vi "Calculate_Trace_Variables.vi"(8 "Baseline":i16, 9 "Threshold":u16, 10 "Peak threshold":i16, 11 "Data in":u16[](array[numeric])) -> (0 "Offset":i16, 1 "Pulse height":i16, 2 "Cut off":i16, 3 "Number of peaks":i16, 4 "Integral":i32, 5 "Data out":u16[](array[numeric]))   [LabVIEW 2013]
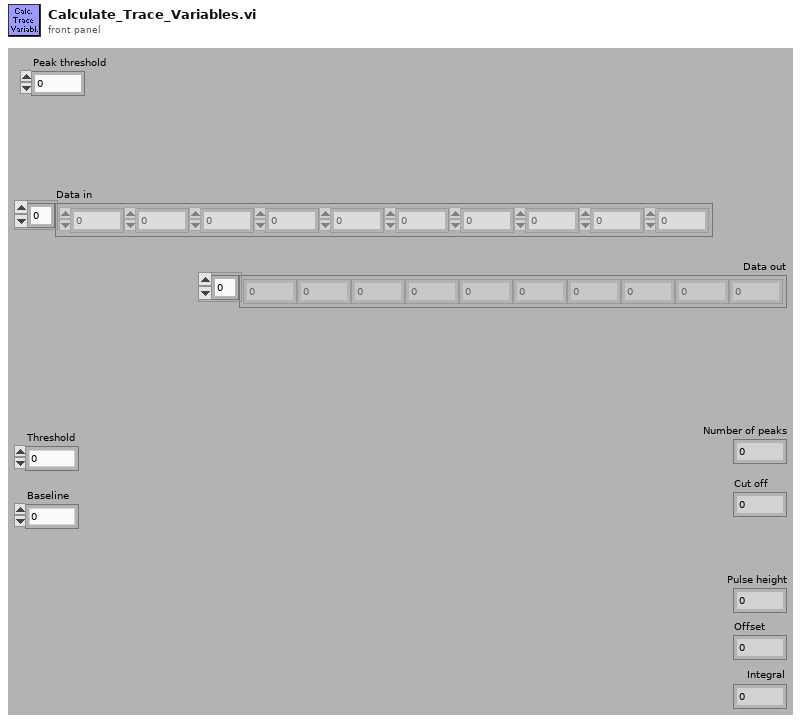
[diagram p1: front panel]
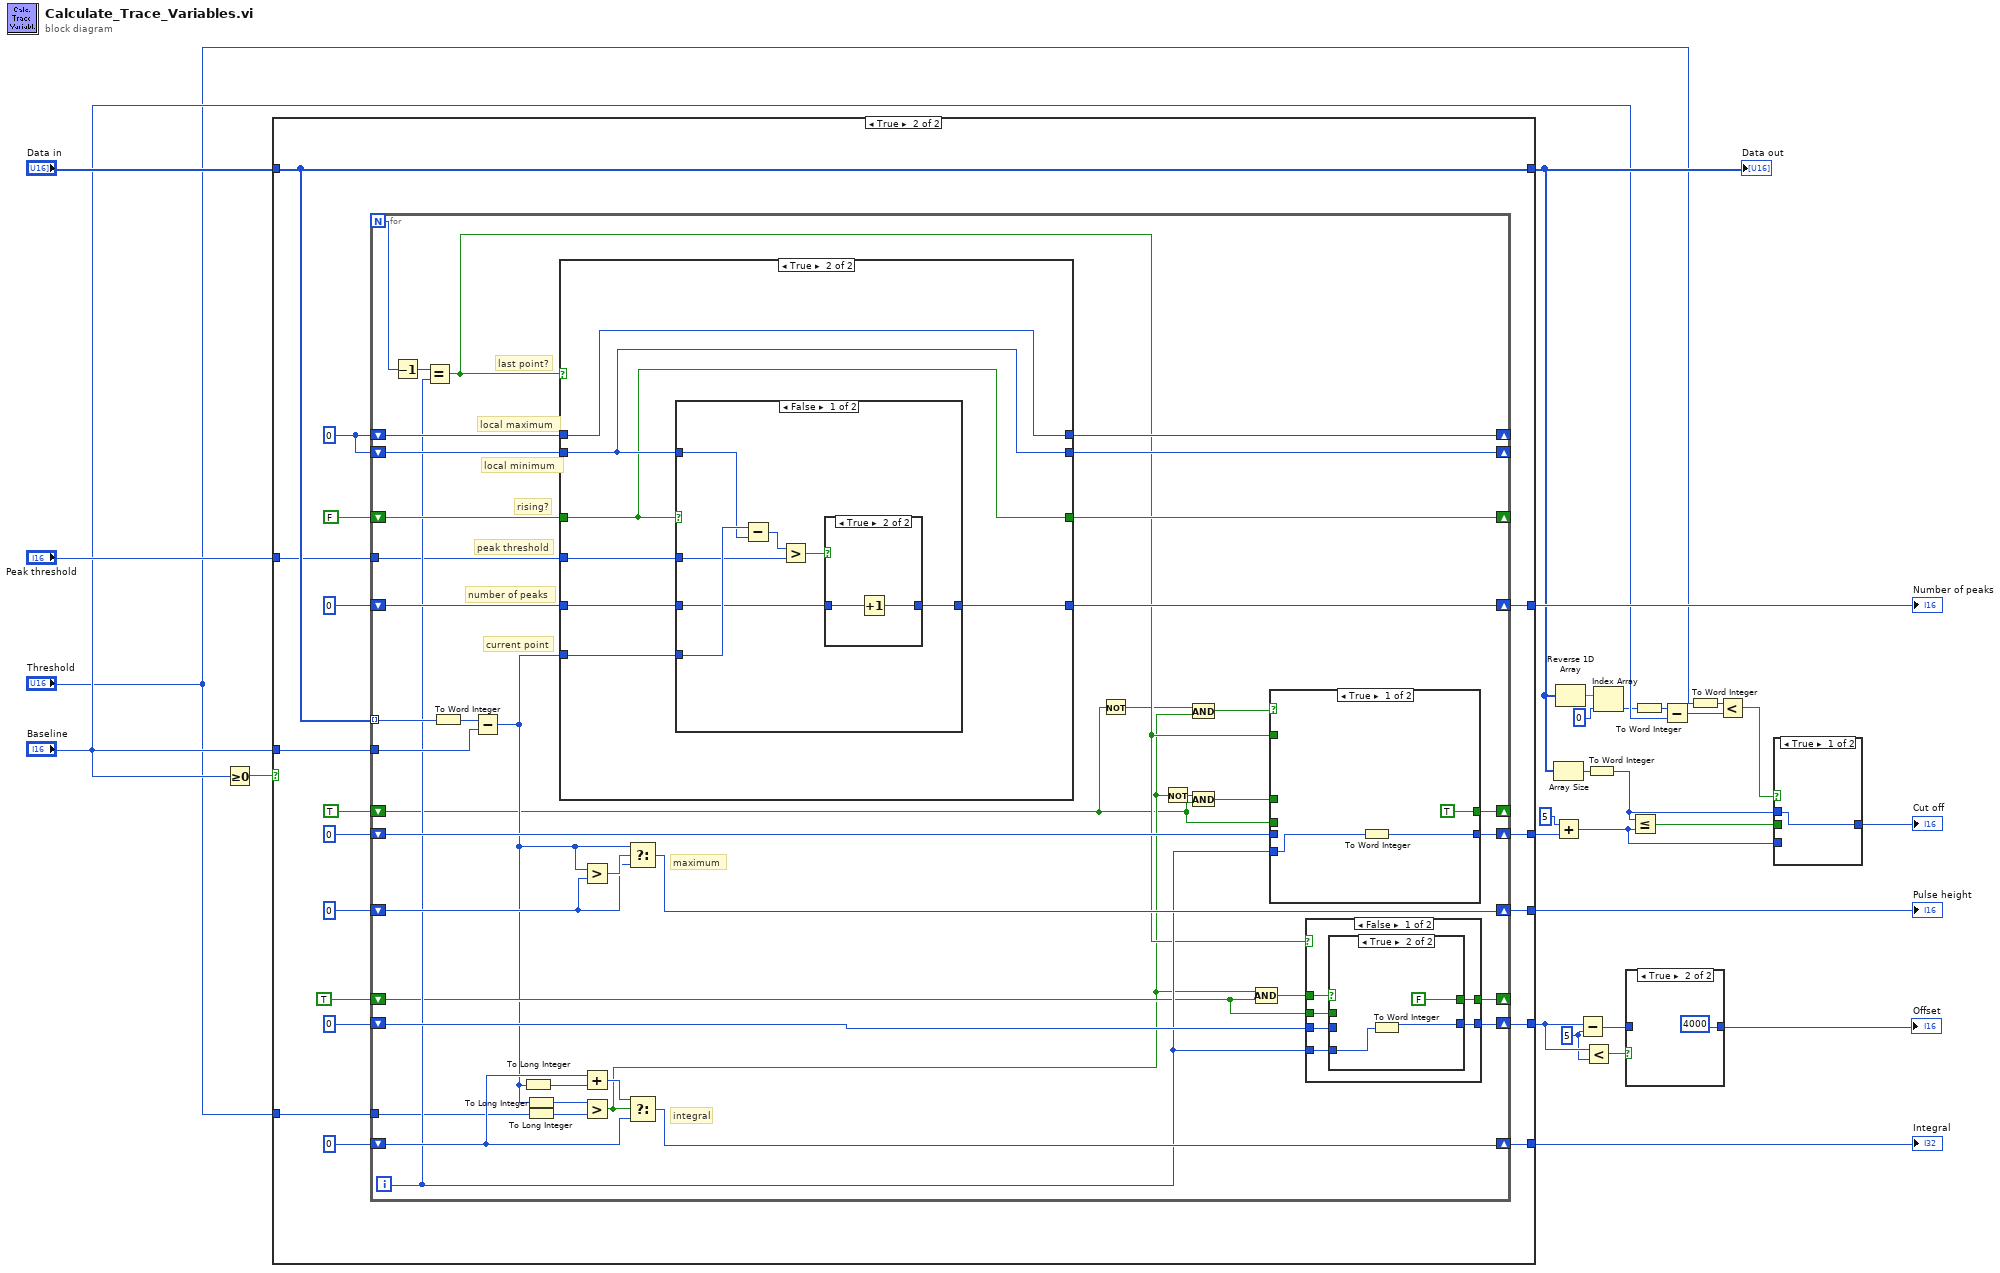
[diagram p0: block diagram]
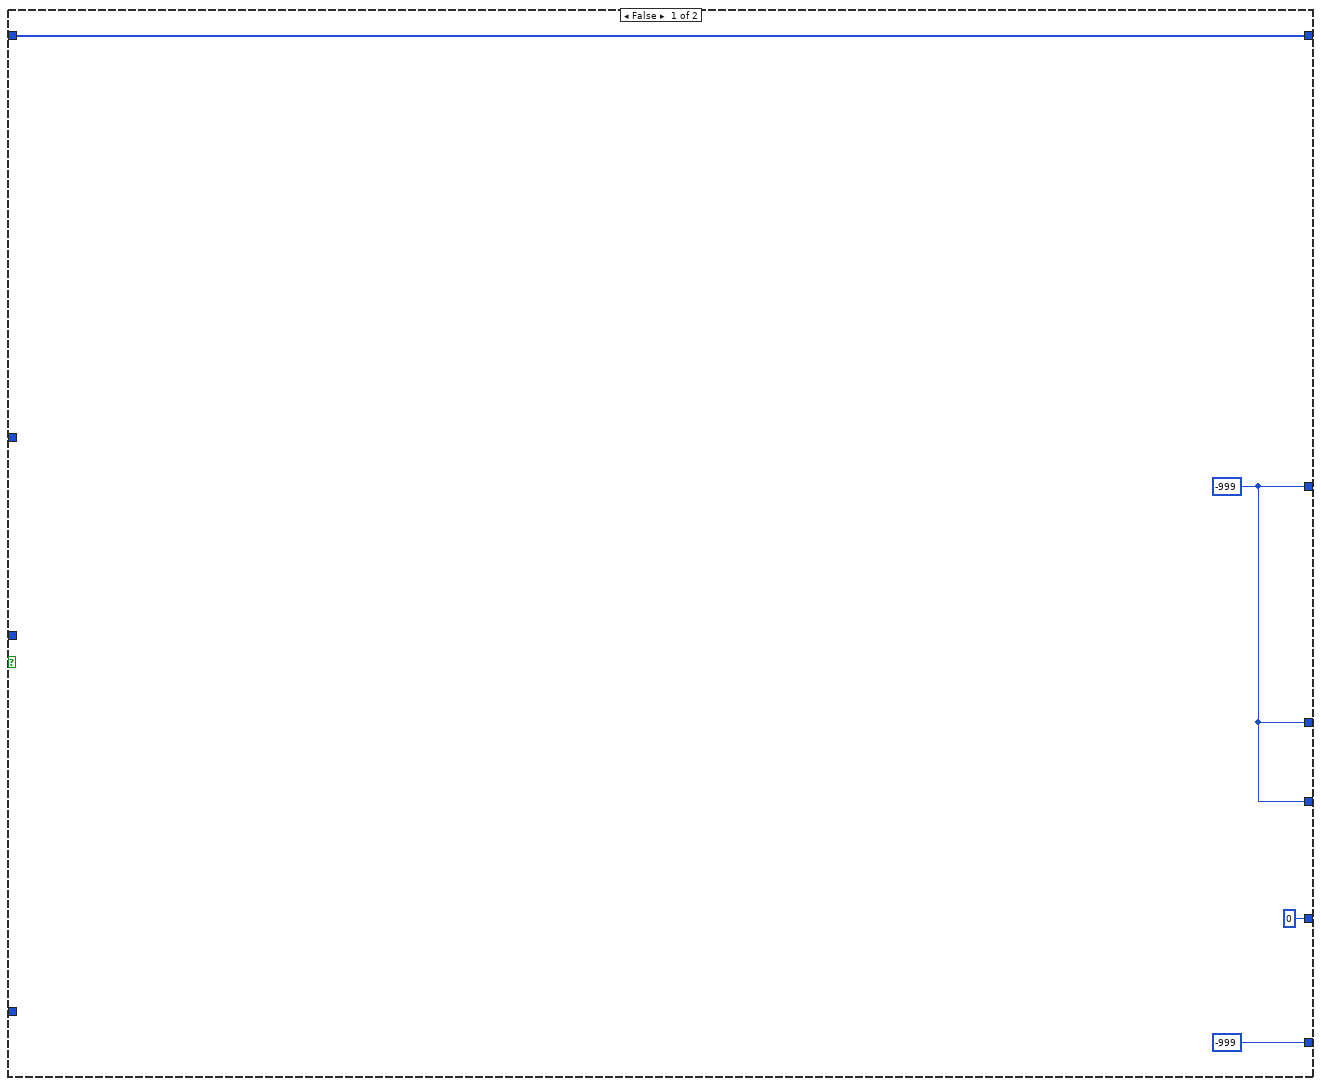
[diagram p5: hidden frame]
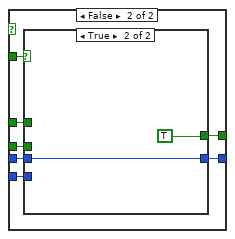
[diagram p6: hidden frame]
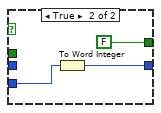
[diagram p8: hidden frame]
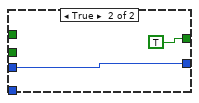
[diagram p10: hidden frame]
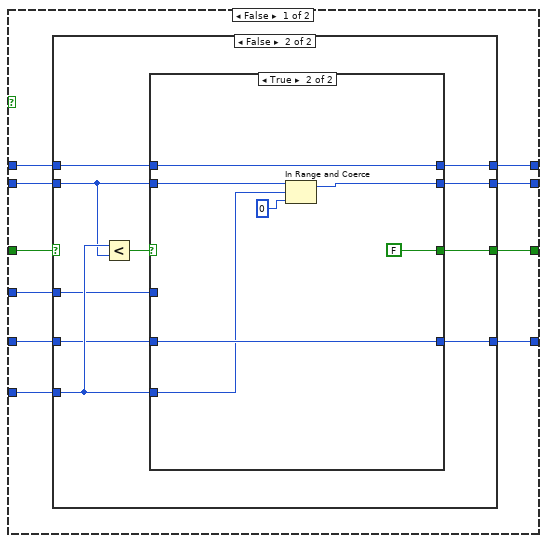
[diagram p11: hidden frame]
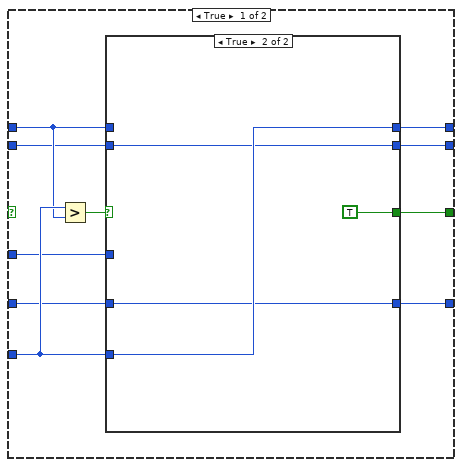
[diagram p12: hidden frame]
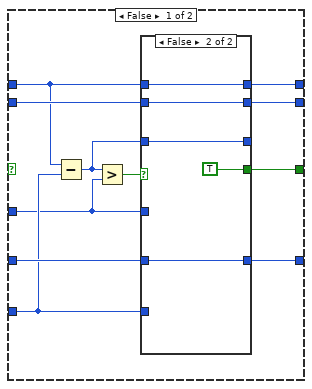
[diagram p13: hidden frame]
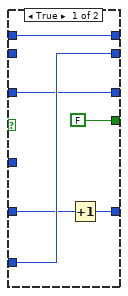
[diagram p14: hidden frame]
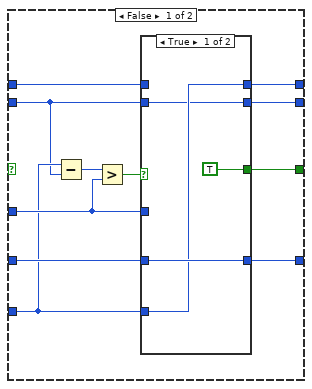
[diagram p15: hidden frame]
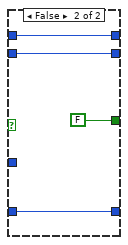
[diagram p16: hidden frame]
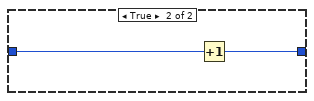
[diagram p18: hidden frame]
diagram:
  w16 = i16 5 ("y")
  n1 = Greater Or Equal To 0?(x="Baseline") -> (x >= 0?=w28:bool)
  n2 = case shown="True" w28 {
    tunnel: "Data in" -> [w32 w50]
    tunnel: [w32 w50] -> w10
    tunnel: [w30 w42] -> w26
    tunnel: [w30 w49] -> w25
    tunnel: [-999 w46] -> w24
    tunnel: "Baseline" -> [_ w48]
    tunnel: "Threshold" -> [_ w34]
    tunnel: [w30 w39] -> w20
    tunnel: [i16 0 w37] -> w17
    tunnel: "Peak threshold" -> [_ w33]
    frame False {
      w30 = i16 -999 ("Number of peaks")
    }
    frame True {
      w45 = i16 0
      n3 = for {
        N -> [w77]
        tunnel: w50 -> [w90] mode=indexing
        shift-right: [w88] -> w49
        shift-left: i16 0 -> [w89]
        tunnel: w48 -> [w86]
        shift-right: [w85] -> w46
        shift-left: 0 -> [w83]
        shift-right: [w78] -> _
        shift-left: w45 -> [w81]
        shift-right: [w74] -> _
        shift-left: w45 -> [w75]
        shift-right: [w79] -> _
        shift-left: FALSE -> [w82]
        shift-right: [w69] -> w42
        shift-left: i16 0 -> [w80]
        tunnel: w34 -> [w52]
        shift-right: [w71] -> w39
        shift-left: i16 0 -> [w70]
        shift-right: [w67] -> w37
        shift-left: i16 0 -> [w65]
        shift-right: [w68] -> _
        shift-left: TRUE -> [w54]
        shift-right: [w61] -> _
        shift-left: TRUE -> [w62]
        tunnel: w33 -> [w53]
        i -> [w64]
        # "last point?"
        # "current point"
        # "number of peaks"
        # "peak threshold"
        # "rising?"
        # "local minimum"
        # "local maximum"
        # "integral"
        # "maximum"
        n4 = Decrement(x=w77) -> (x-1=w76:i32)
        n5 = Equal?(x=w76, y=w64) -> (x = y?=w60:bool)
        n6 = To Word Integer(number=w90) -> (16bit integer=w87:i16)
        n7 = Subtract(x=w87, y=w86) -> (x-y=w59:i16)
        n8 = To Long Integer(number=w59) -> (32bit integer=w73:i32)
        n9 = To Long Integer(number=w59) -> (32bit integer=w58:i32)
        n10 = To Long Integer(number=w52) -> (32bit integer=w51:i32)
        n11 = case shown="True" w60 {
          tunnel: w82 -> [w137 w210]
          tunnel: w81 -> [w136 w212]
          tunnel: w75 -> [w135 w211]
          tunnel: w59 -> [w134 w214]
          tunnel: w53 -> [w133 w213]
          tunnel: w80 -> [w132 w215]
          tunnel: [w131 w216] -> w69
          tunnel: [w130 w210] -> w79
          tunnel: [w129 w211] -> w74
          tunnel: [w128 w212] -> w78
          frame False {
            n12 = case shown="False" w137 {
              tunnel: w136 -> [w145 w174]
              tunnel: w135 -> [w139 w175]
              tunnel: w134 -> [w146 w182]
              tunnel: w133 -> [w144 w181]
              tunnel: w132 -> [w143 w180]
              tunnel: [w142 w179] -> w131
              tunnel: [w141 w178] -> w130
              tunnel: [w140 w177] -> w129
              tunnel: [w138 w176] -> w128
              frame True {
                n13 = Greater?(x=w146, y=w145) -> (0:w147:bool)
                n14 = case shown="True" w147 {
                  tunnel: w146 -> [w154 w173]
                  tunnel: w145 -> [w150 _]
                  tunnel: w144 -> [w149 _]
                  tunnel: w143 -> [w157 w171]
                  tunnel: [w156 w171] -> w142
                  tunnel: [w155 TRUE] -> w141
                  tunnel: [w153 w172] -> w140
                  tunnel: w139 -> [w152 w172]
                  tunnel: [w151 w173] -> w138
                  frame False {
                    n15 = Subtract(x=w150, y=w154) -> (x-y=w148:i16)
                    n16 = Greater?(x=w148, y=w149) -> (0:w158:bool)
                    n17 = case shown="False" w158 {
                      tunnel: w157 -> [w161 w168]
                      tunnel: [w160 w168] -> w156
                      tunnel: [FALSE TRUE] -> w155
                      tunnel: w154 -> [w163 _]
                      tunnel: [w163 w167] -> w153
                      tunnel: w152 -> [_ w167]
                      tunnel: [w162 w166] -> w151
                      tunnel: w150 -> [w162 w166]
                      tunnel: w149 -> [_ _]
                      tunnel: [w159 w165] -> _
                      tunnel: w148 -> [w159 w165]
                      frame True {
                        n18 = Increment(x=w161) -> (x+1=w160:i16)
                      }
                      frame False {
                      }
                    }
                  }
                  frame True {
                  }
                }
              }
              frame False {
                n19 = Less?(x=w182, y=w175) -> (x < y?=w183:bool)
                n20 = case shown="True" w183 {
                  tunnel: w182 -> [w186 w205]
                  tunnel: w174 -> [w184 w208]
                  tunnel: w181 -> [w187 _]
                  tunnel: w180 -> [w192 w209]
                  tunnel: [w191 w209] -> w179
                  tunnel: [w190 FALSE] -> w178
                  tunnel: [w189 w206] -> w177
                  tunnel: w175 -> [w185 w207]
                  tunnel: [w188 w208] -> w176
                  frame False {
                    n21 = Subtract(x=w186, y=w185) -> (x-y=w194:i16)
                    n22 = Greater?(x=w194, y=w187) -> (0:w193:bool)
                    n23 = case shown="True" w193 {
                      tunnel: w192 -> [w197 w201]
                      tunnel: [w197 w201] -> w191
                      tunnel: [TRUE FALSE] -> w190
                      tunnel: w186 -> [w196 _]
                      tunnel: [w195 w200] -> w189
                      tunnel: w185 -> [w195 w200]
                      tunnel: [w196 w199] -> w188
                      tunnel: w184 -> [_ w199]
                      tunnel: w187 -> [_ _]
                      frame True {
                      }
                      frame False {
                      }
                    }
                  }
                  frame True {
                    n24 = In Range and Coerce(upper limit=w207, x=w205, lower limit=i16 0) -> (coerced(x)=w206:i16)  [unwired: 1 out]
                  }
                }
              }
            }
          }
          frame True {
            n25 = case shown="False" w210 {
              tunnel: [w218 w227] -> w216
              tunnel: w215 -> [w219 w228]
              tunnel: w214 -> [w223 _]
              tunnel: w211 -> [w217 _]
              tunnel: w213 -> [w222 _]
              frame False {
                n26 = Subtract(x=w223, y=w217) -> (x-y=w221:i16)
                n27 = Greater?(x=w221, y=w222) -> (0:w220:bool)
                n28 = case shown="True" w220 {
                  tunnel: w219 -> [w224 w226]
                  tunnel: [w224 w225] -> w218
                  frame False {
                  }
                  frame True {
                    n29 = Increment(x=w226) -> (x+1=w225:i16)
                  }
                }
              }
              frame True {
                n30 = Increment(x=w228) -> (x+1=w227:i16)
              }
            }
          }
        }
        n31 = Greater?(x=w59, y=w89) -> (0:w91:bool)
        n32 = Add(x=w83, y=w73) -> (x+y=w84:i32)
        n33 = Greater?(x=w58, y=w51) -> (0:w57:bool)
        n34 = Select(t=w59, s=w91, f=w89) -> (s? t:f=w88:i16)
        n35 = Select(t=w84, s=w57, f=w83) -> (s? t:f=w85:i32)
        n36 = Not(x=w54) -> (.not. x?=w55:bool)
        n37 = Not(x=w57) -> (.not. x?=w63:bool)
        n38 = Compound Arithmetic op=AND(w55, w57) -> (w56:bool)
        n39 = Compound Arithmetic op=AND(w63, w54) -> (w72:bool)
        n40 = Compound Arithmetic op=AND(w57, w62) -> (w66:bool)
        n41 = case shown="True" w56 {
          tunnel: w72 -> [_ w101]
          tunnel: [w92 w100] -> w71
          tunnel: w70 -> [_ w99]
          tunnel: [TRUE ("First time") w98] -> w68
          tunnel: w54 -> [_ w97]
          tunnel: w64 -> [w93 w96]
          tunnel: w60 -> [_ w95]
          frame True {
            n42 = To Word Integer(number=w93) -> (16bit integer=w92:i16)
          }
          frame False {
            n43 = case shown="True" w95 {
              tunnel: w101 -> [w107 _]
              tunnel: [w103 w114] -> w100
              tunnel: w99 -> [w105 w114]
              tunnel: w96 -> [w104 _]
              tunnel: [w102 TRUE] -> w98
              tunnel: w97 -> [w106 _]
              frame False {
                n44 = case shown="False" w107 {
                  tunnel: w104 -> [_ w111]
                  tunnel: [w109 w112] -> w103
                  tunnel: w105 -> [w109 _]
                  tunnel: [w108 FALSE ("First time")] -> w102
                  tunnel: w106 -> [w108 _]
                  frame False {
                  }
                  frame True {
                    n45 = To Word Integer(number=w111) -> (16bit integer=w112:i16)
                  }
                }
              }
              frame True {
              }
            }
          }
        }
        n46 = case shown="False" w60 {
          tunnel: [w115 w126] -> w67
          tunnel: w66 -> [w120 _]
          tunnel: w65 -> [w118 w126]
          tunnel: w64 -> [w117 _]
          tunnel: w62 -> [w119 _]
          tunnel: [w116 TRUE] -> w61
          frame False {
            n47 = case shown="True" w120 {
              tunnel: w117 -> [_ w124]
              tunnel: [w122 w125] -> w115
              tunnel: w118 -> [w122 _]
              tunnel: w119 -> [w121 _]
              tunnel: [w121 FALSE] -> w116
              frame False {
              }
              frame True {
                n48 = To Word Integer(number=w124) -> (16bit integer=w125:i16)
              }
            }
          }
          frame True {
          }
        }
      }
    }
  }
  "Data out" <- w10
  "Number of peaks" <- w26
  "Pulse height" <- w25
  "Integral" <- w24
  n49 = Array Size(array=w10) -> (size(s)=w13:i32)
  n50 = Add(x=i16 5, y=w20) -> (x+y=w14:i16)
  n51 = Reverse 1D Array(array=w10) -> (reversed array=w9:u16[])
  n52 = Subtract(x=w17, y=w16) -> (x-y=w21:i16)
  n53 = Less?(x=w17, y=w16) -> (x < y?=w23:bool)
  n54 = To Word Integer(number=w13) -> (16bit integer=w12:i16)
  n55 = Index Array(array=w9, index=0) -> (element=w4:u16)
  n56 = case shown="True" w23 {
    tunnel: w21 -> [w229 _]
    tunnel: [w229 i16 4000 ("Number of peaks")] -> w22
    frame False {
    }
    frame True {
    }
  }
  "Offset" <- w22
  n57 = Less Or Equal?(x=w12, y=w14) -> (x <= y?=w11:bool)
  n58 = To Word Integer(number=w4) -> (16bit integer=w5:i16)
  n59 = Subtract(x=w5, y="Baseline") -> (x-y=w3:i16)
  n60 = To Word Integer(number="Threshold") -> (16bit integer=w1:i16)
  n61 = Less?(x=w1, y=w3) -> (x < y?=w7:bool)
  n62 = case shown="True" w7 {
    tunnel: [w231 w235] -> w15
    tunnel: w14 -> [_ w234]
    tunnel: w12 -> [w231 w233]
    tunnel: w11 -> [_ w232]
    frame True {
    }
    frame False {
      n63 = case shown="True" w232 {
        tunnel: w233 -> [_ w237]
        tunnel: [w236 w237] -> w235
        tunnel: w234 -> [w236 _]
        frame False {
        }
        frame True {
        }
      }
    }
  }
  "Cut off" <- w15
